vi "Set Value.vi"(8 "error in (no error)":errorcluster, 10 "Value":variant, 11 "Cell Context in":refnum<class "Cell Context.lvclass">) -> (0 "error out":errorcluster, 3 "Cell Context out":refnum<class "Cell Context.lvclass">)   [LabVIEW 2023, in "SourceGrid.lvlib" / "Cell Context.lvclass"]
uses:
  Cell Context.lvclass
  Cell Context.lvclass/Cell Context.ctl
  D:/git/Sourcegrid-LabVIEW/dll/SourceGrid.dll
  dll/SourceGrid.dll
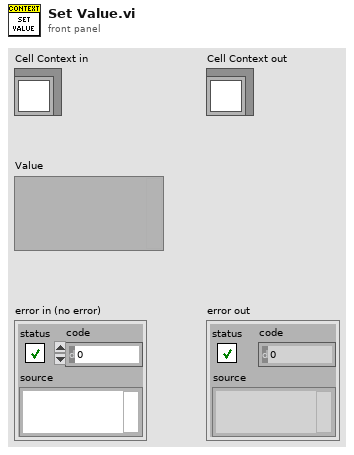
[diagram p1: front panel]
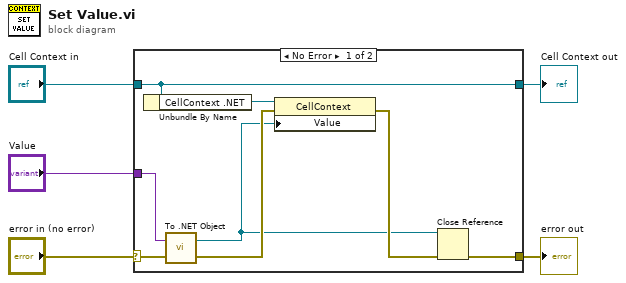
[diagram p0: block diagram]
diagram:
  n1 = case shown="No Error" "error in (no error)" {
    selector: "error in (no error)" -> [w12 w14]
    tunnel: [w7 w14] -> w4
    tunnel: [w10 w15] -> w2
    tunnel: "Cell Context in" -> [w10 w15]
    tunnel: "Value" -> [w13 _]
    frame No Error {
      n2 = Unbundle By Name(w10) -> ("CellContext .NET"=w11:refnum<k24>)
      n3 = call <vilib>:"To .NET Object.vi"("error in (no error)"=w12, "anything"=w13) -> ("error out"=w9:errorcluster, ".NET object"=w6:refnum<k24>)
      n4 = property class="CellContext"(reference=w11, error in=w9, "Value"=w6) -> (error out=w8:errorcluster)  [unwired: 1 out]
      n5 = Close Reference(reference=w6, error in (no error)=w8) -> (error out=w7:errorcluster)
    }
    frame Error {
    }
  }
  "error out" <- w4
  "Cell Context out" <- w2
